vi "Auto_Routine_BlueRightTwoPieceTRAJ.vi"   [LabVIEW 2023]
uses:
  Arm2/ArmGetSetpointEnum.ctl
  Trajectory/TrajectoryGlobals.vi
  <vilib>/Rock Robotics/WPI/ThirdParty/JAS_Junk/TrajLib/Trajectory_Library.lvlib
types:
  T1 = typedef "ArmGetSetpointEnum.ctl" = enum16{"ArmFloorPickup", "ArmAmpDeposit", "ArmSpeakerShoot", "ArmStartPosition", "ArmRestPosition", "ArmSourceIntake", "ArmAwayShoot"}
  T2 = typedef "Trajectory_Library.lvlib/TRAJECTORY.ctl" = cluster{"TotalTImeSecs":dbl, "States":T3[]}
  T3 = typedef "Trajectory_Library.lvlib/TRAJ_STATE.ctl" = cluster{"TimeSeconds":dbl, "Velocity":dbl, "Acceleration":dbl, "POSE":T4, "Curvature":dbl}
  T4 = typedef "Trajectory_Library.lvlib/POSE2D.ctl" = cluster{"TRANSLATION":T5, "ROTATION":T6}
  T5 = typedef "Trajectory_Library.lvlib/TRANSLATION2D.ctl" = cluster{"X":dbl, "Y":dbl}
  T6 = typedef "Trajectory_Library.lvlib/ROTATION2D.ctl" = cluster{"VALUE":dbl, "COS":dbl, "SIN":dbl}
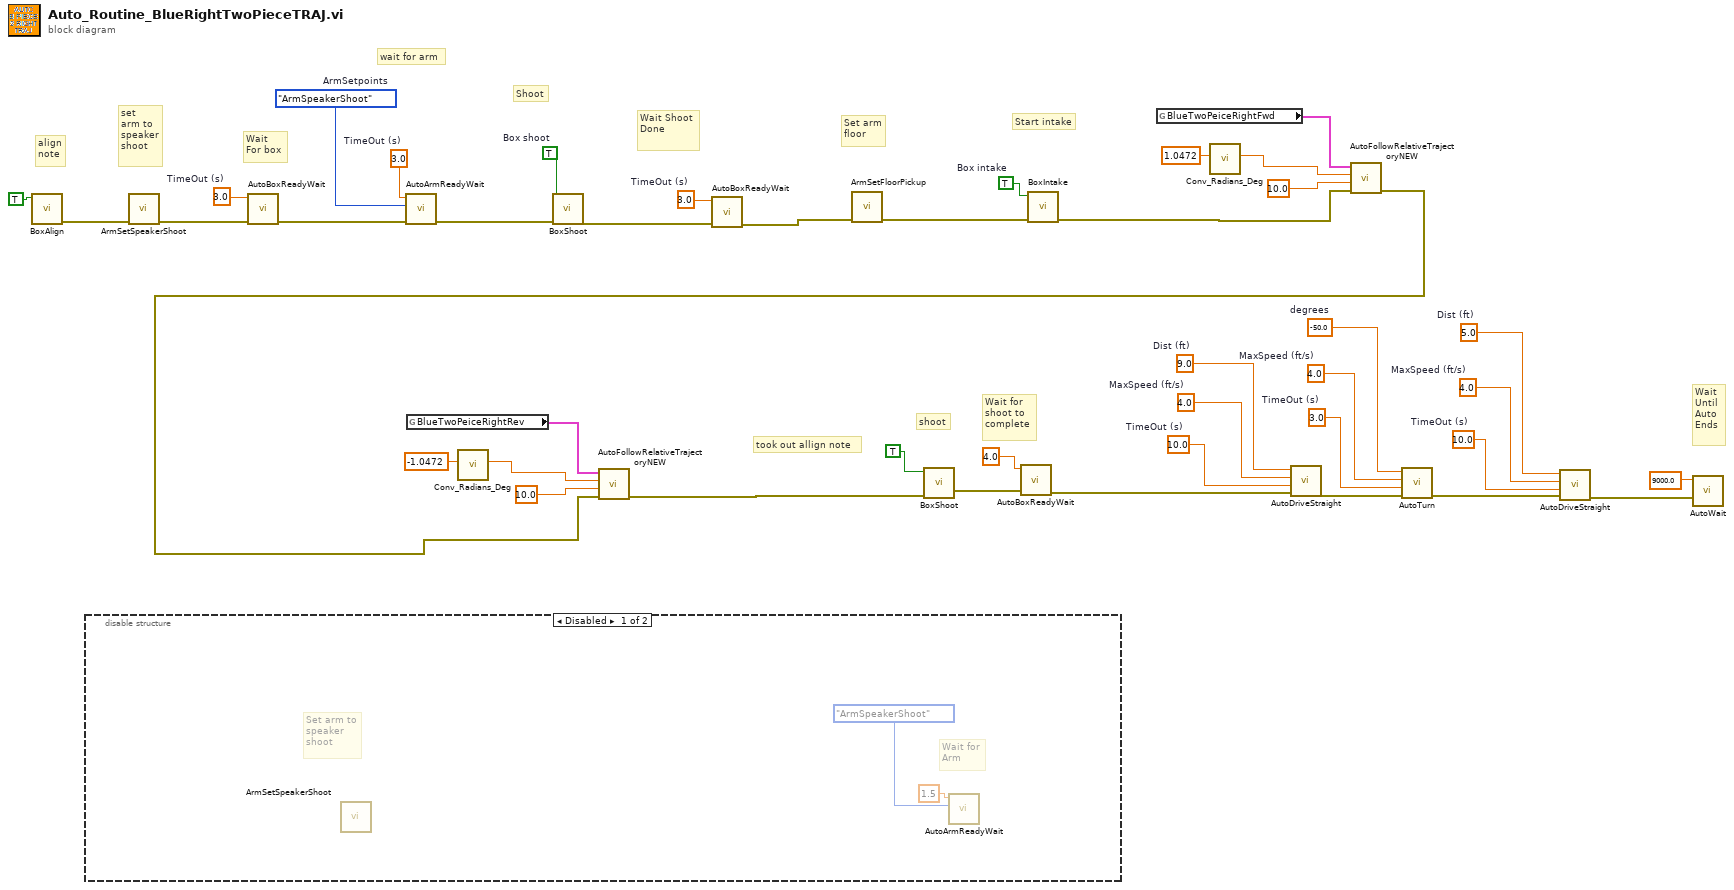
[diagram p0: block diagram]
diagram:
  w3 = -50.0  # degrees
  w4 = 4.0  # MaxSpeed (ft/s)
  w5 = 3.0  # TimeOut (s)
  w9 = 5.0  # Dist (ft)
  w10 = 4.0  # MaxSpeed (ft/s)
  w11 = 10.0  # TimeOut (s)
  w12 = 9.0  # Dist (ft)
  w13 = 4.0  # MaxSpeed (ft/s)
  w14 = 10.0  # TimeOut (s)
  w32 = 3.0  # TimeOut (s)
  w42 = TRUE  # Box intake
  w41 = TRUE  # Box shoot
  w40 = ArmGetSetpointEnum."ArmSpeakerShoot"  # ArmSetpoints
  w39 = 3.0  # TimeOut (s)
  w35 = 3.0  # TimeOut (s)
  # "took out allign note"
  # "Wait\nUntil\nAuto \nEnds"
  # "Wait for\nshoot to\ncomplete"
  # "shoot"
  # "Start intake"
  # "Set arm\nfloor"
  # "Wait Shoot\nDone"
  # "Shoot"
  # "Wait\nFor box"
  # "set \narm to\nspeaker\nshoot"
  # "align\nnote"
  # "wait for arm"
  n1 = call "BoxAlign.vi"("box align"=TRUE) -> ("error out"=w33:errorcluster)  [unwired: 10 in]
  n2 = disable-structure shown="Disabled" {
    frame Disabled {
      # "Wait for\nArm"
      # "Set arm to\nspeaker \nshoot"
      n3 = call "ArmSetSpeakerShoot.vi"() -> ()  [unwired: 11 in, 1 out]
      n4 = call "AutoArmReadyWait.vi"("ArmSetpoints"=ArmGetSetpointEnum."ArmSpeakerShoot", "TimeOut (s)"=1.5) -> ("error out"=w44:errorcluster, "error in (no error)"=w43:errorcluster)  [unwired: 8 in]
    }
    frame Enabled {
    }
  }
  n5 = call "ArmSetSpeakerShoot.vi"("error in (no error)"=w33) -> ("error out"=w31:errorcluster)  [unwired: 10 in]
  n6 = call "AutoBoxReadyWait.vi"("error in (no error)"=w31, "TimeOut (s)"=w32) -> ("error out"=w30:errorcluster)  [unwired: 9 in]
  n7 = call "AutoArmReadyWait.vi"("error in (no error)"=w30, "ArmSetpoints"=w40, "TimeOut (s)"=w39) -> ("error out"=w36:errorcluster)  [unwired: 8 in]
  n8 = global read "TrajectoryGlobals.vi" "BlueTwoPeiceRightRev"() -> (w19:T2)
  n9 = call <vilib>:"Conv_Radians_Deg.vi"("Radians"=-1.0472) -> ("Degrees"=w17:dbl)  [unwired: 10 in]
  n10 = call "BoxShoot.vi"("error in (no error)"=w36, "Box shoot"=w41) -> ("error out"=w37:errorcluster)  [unwired: 9 in]
  n11 = call "AutoBoxReadyWait.vi"("error in (no error)"=w37, "TimeOut (s)"=w35) -> ("error out"=w29:errorcluster)  [unwired: 9 in]
  n12 = call "ArmSetFloorPickup.vi"("error in (no error)"=w29) -> ("error out"=w38:errorcluster)  [unwired: 10 in]
  n13 = call "BoxIntake.vi"("error in (no error)"=w38, "Box intake"=w42) -> ("error out"=w28:errorcluster)  [unwired: 9 in]
  n14 = global read "TrajectoryGlobals.vi" "BlueTwoPeiceRightFwd"() -> (w27:T2)
  n15 = call <vilib>:"Conv_Radians_Deg.vi"("Radians"=1.0472) -> ("Degrees"=w25:dbl)  [unwired: 10 in]
  n16 = call "AutoFollowRelativeTrajectoryNEW.vi"("error in (no error)"=w28, "TimeOut (s)"=10.0, "End Orientation"=w25, "Trajectory"=w27) -> ("error out"=w2:errorcluster)  [unwired: 7 in]
  n17 = call "AutoFollowRelativeTrajectoryNEW.vi"("error in (no error)"=w2, "TimeOut (s)"=10.0, "End Orientation"=w17, "Trajectory"=w19) -> ("error out"=w1:errorcluster)  [unwired: 7 in]
  n18 = call "BoxShoot.vi"("error in (no error)"=w1, "Box shoot"=TRUE) -> ("error out"=w22:errorcluster)  [unwired: 9 in]
  n19 = call "AutoBoxReadyWait.vi"("error in (no error)"=w22, "TimeOut (s)"=4.0) -> ("error out"=w15:errorcluster)  [unwired: 9 in]
  n20 = call "AutoDriveStraight.vi"("error in (no error)"=w15, "TimeOut (s)"=w14, "MaxSpeed (ft/s)"=w13, "Dist (ft)"=w12) -> ("error out"=w6:errorcluster)  [unwired: 7 in]
  n21 = call "AutoTurn.vi"("error in (no error)"=w6, "TimeOut (s)"=w5, "MaxSpeed (ft/s)"=w4, "degrees"=w3) -> ("error out"=w8:errorcluster)  [unwired: 7 in]
  n22 = call "AutoDriveStraight.vi"("error in (no error)"=w8, "TimeOut (s)"=w11, "MaxSpeed (ft/s)"=w10, "Dist (ft)"=w9) -> ("error out"=w7:errorcluster)  [unwired: 7 in]
  n23 = call "AutoWait.vi"("error in (no error)"=w7, "TimeOut (s)"=9000.0) -> ()  [unwired: 9 in, 1 out]
